vi "Create (From State String Constant).vi"(8 "error in (no error)":errorcluster, 10 "State String Constant":refnum<vi>) -> (0 "error out":errorcluster, 1 "Structure Found in":refnum<vi>, 2 "Found JKI SMs?":bool, 3 "JKI SM out":refnum<class "JKI SM.lvclass">)   [LabVIEW 2013, in "JKI State Machine API.lvlib" / "JKI SM.lvclass"]
uses:
  JKI SM.lvclass
  JKI State Machine API.lvlib
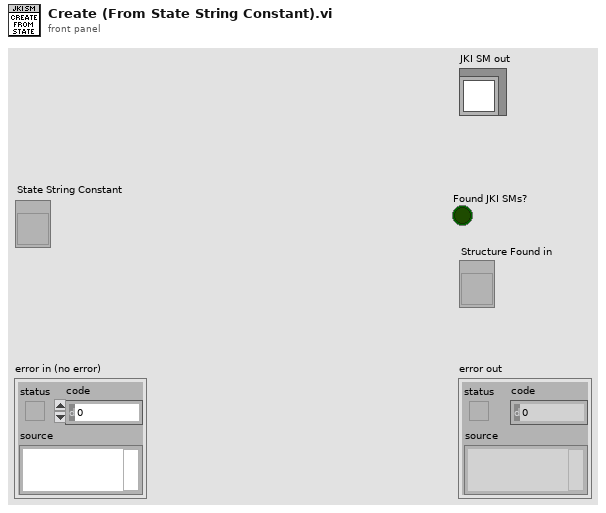
[diagram p1: front panel]
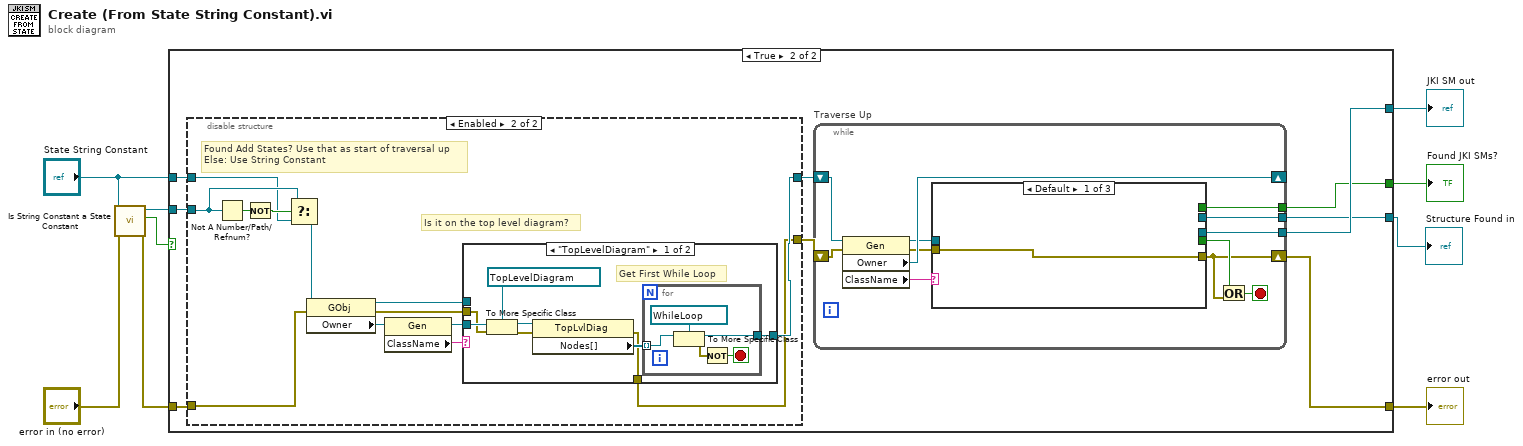
[diagram p0: block diagram]
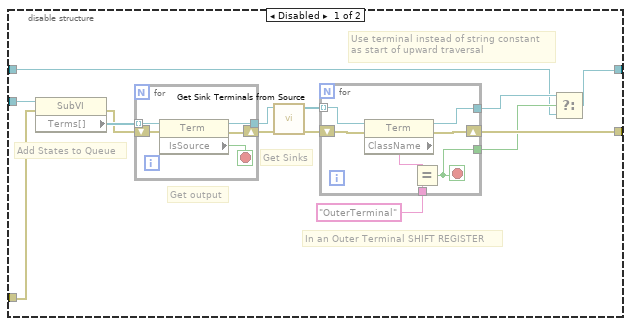
[diagram p3: hidden frame]
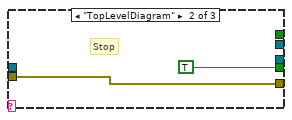
[diagram p5: hidden frame]
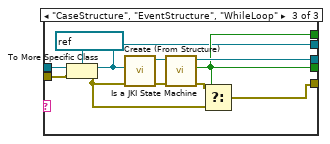
[diagram p6: hidden frame]
diagram:
  n1 = call "Is String Constant a State Constant.vi"("error in (no error)"="error in (no error)", "GObj Refnum"="State String Constant") -> ("error out"=w3:errorcluster, "Is States Constant"=w2:bool, "Add States to Queue"=w4:refnum<vi>)  [unwired: 7 in]
  n2 = case shown="True" w2 {
    tunnel: [w10 w18] -> w9
    tunnel: [_ w19] -> w8
    tunnel: "State String Constant" -> [_ w14]
    tunnel: [_ w17] -> w5
    tunnel: w4 -> [_ w16]
    tunnel: w3 -> [w10 w12]
    tunnel: [_ w11] -> w1
    frame False {
    }
    frame True {
      n3 = disable-structure shown="Enabled" {
        disable-tunnel: w16 -> [w33 w56]
        disable-tunnel: [w26 w49] -> w15
        disable-tunnel: w14 -> [w22 w55]
        disable-tunnel: [w21 w52] -> w13
        disable-tunnel: w12 -> [w20 w50]
        frame Disabled {
          # "Use terminal instead of string constant\nas start of upward traversal"
          # "In an Outer Terminal SHIFT REGISTER"
          # "Get Sinks"
          # "Get output"
          # "Add States to Queue"
          n4 = property class="SubVI"(reference=w33, error in=w20) -> (error out=w31:errorcluster, "Terms[]"=w32:refnum<vi>[])  [unwired: 1 out]
          n5 = for {
            tunnel: w32 -> [w45] mode=indexing
            shift-right: [w43] -> w29
            shift-left: w31 -> [w44]
            tunnel: [w41] -> w30
            stop <- w42 stop-if-true
            n6 = property class="Term"(reference=w45, error in=w44) -> (reference out=w41:refnum<vi>, error out=w43:errorcluster, "IsSource"=w42:bool)
          }
          n7 = call "Get Sink Terminals from Source.vi"("error in (no error)"=w29, "Source Terminal"=w30) -> ("error out"=w27:errorcluster, "Sink Terminals"=w28:refnum<vi>[])  [unwired: 8 in]
          n8 = for {
            tunnel: w28 -> [w40] mode=indexing
            tunnel: "OuterTerminal" ("Class Name") -> [w37]
            tunnel: [w35] -> w23
            tunnel: [w34] -> w24
            shift-right: [w38] -> w26
            shift-left: w27 -> [w39]
            stop <- w34 stop-if-true
            n9 = property class="Term"(reference=w40, error in=w39) -> (reference out=w35:refnum<vi>, error out=w38:errorcluster, "ClassName"=w36:string)
            n10 = Equal?(x=w36, y=w37) -> (x = y?=w34:bool)
          }
          n11 = Select(t=w23, s=w24, f=w22) -> (s? t:f=w21:refnum<vi>)
        }
        frame Enabled {
          # "Is it on the top level diagram?"
          # "Found Add States? Use that as start of traversal up\nElse: Use String Constant"
          n12 = Not A Number/Path/Refnum?(number/path/refnum=w56) -> (NaN/Path/Refnum?=w58:bool)
          n13 = Not(x=w58) -> (.not. x?=w57:bool)
          n14 = Select(t=w56, s=w57, f=w55) -> (s? t:f=w53:refnum<vi>)
          n15 = property class="GObj"(reference=w53, error in=w50) -> (reference out=w54:refnum<vi>, error out=w51:errorcluster, "Owner"=w47:refnum<vi>)
          n16 = property class="Gen"(reference=w47) -> (reference out=w46:refnum<vi>, "ClassName"=w48:string)  [unwired: 1 in, 1 out]
          n17 = case shown="\"TopLevelDiagram\"" w48 {
            tunnel: w54 -> [_ w73]
            tunnel: w46 -> [w66 _]
            tunnel: [w62 w73] -> w52
            tunnel: w51 -> [w60 w72]
            tunnel: [w59 w72] -> w49
            frame "TopLevelDiagram" {
              # "Get First While Loop"
              n18 = To More Specific Class(target class=refnum<vi> refnum ("Owner"), reference=w66, error in=w60) -> (specific class reference=w64:refnum<vi>, error out=w61:errorcluster)
              n19 = property class="TopLvlDiag"(reference=w64, error in=w61) -> (error out=w59:errorcluster, "Nodes[]"=w63:refnum<vi>[])  [unwired: 1 out]
              n20 = for {
                tunnel: w63 -> [w71] mode=indexing
                tunnel: [w68] -> w62
                stop <- w67 stop-if-true
                n21 = To More Specific Class(target class=refnum<vi> refnum ("Owner"), reference=w71) -> (specific class reference=w68:refnum<vi>, error out=w69:errorcluster)  [unwired: 1 in]
                n22 = Not(x=w69) -> (.not. x?=w67:bool)
              }
            }
            frame Default {
            }
          }
        }
      }
      n23 = while "Traverse Up" {
        shift-right: [w85] -> _
        shift-left: w13 -> [w84]
        shift-right: [w76] -> w18
        shift-left: w15 -> [w80]
        tunnel: [w79] -> w19
        tunnel: [w75] -> w17
        tunnel: [w74] -> w11
        stop <- w78 stop-if-true
        n24 = property class="Gen"(reference=w84, error in=w80) -> (reference out=w82:refnum<vi>, error out=w81:errorcluster, "Owner"=w85:refnum<vi>, "ClassName"=w83:string)
        n25 = case shown="Default" w83 {
          tunnel: w82 -> [_ _ w99]
          tunnel: [w86 w88 w91] -> w76
          tunnel: w81 -> [w86 w88 w97]
          tunnel: [_ _ w95] -> w79
          tunnel: [_ TRUE ("Is a JKI State Machine") w90] -> w77
          tunnel: [_ _ w90] -> w75
          tunnel: [_ _ w89] -> w74
          frame Default {
          }
          frame "TopLevelDiagram" {
            # "Stop"
          }
          frame "CaseStructure", "EventStructure", "WhileLoop" {
            n26 = To More Specific Class(target class=refnum<vi> refnum ("Structure"), reference=w99, error in=w97) -> (specific class reference=w89:refnum<vi>, error out=w92:errorcluster)
            n27 = call "Create (From Structure).vi"("error in (no error)"=w92, "Structure"=w89) -> ("error out"=w94:errorcluster, "JKI SM out"=w96:refnum<class "JKI SM.lvclass">)  [unwired: 8 in]
            n28 = call "Is a JKI State Machine.vi"("error in (no error)"=w94, "JKI SM in"=w96) -> ("error out"=w93:errorcluster, "Is a JKI State Machine"=w90:bool, "JKI SM out"=w95:refnum<class "JKI SM.lvclass">)  [unwired: 7 in]
            n29 = Select(t=w93, s=w90, f=w92) -> (s? t:f=w91:errorcluster)
          }
        }
        n30 = Or(x=w77, y=w76) -> (x .or. y?=w78:bool)
      }
    }
  }
  "error out" <- w9
  "JKI SM out" <- w8
  "Found JKI SMs?" <- w5
  "Structure Found in" <- w1
